vi "Test ACME SubTest.vi"(8 "error in (no error)":errorcluster, 11 "Label (VI Title)":string) -> (0 "error out":errorcluster)   [LabVIEW 2020]
uses:
  classes/Test/Test.lvclass
  Assert.ACME.lvclass
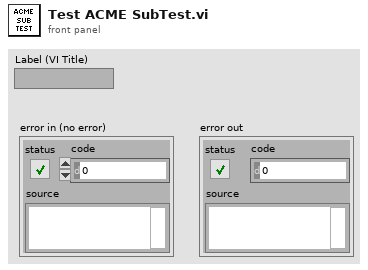
[diagram p1: front panel]
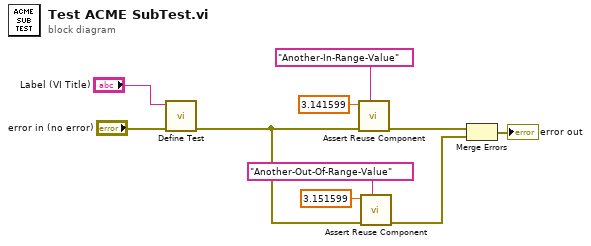
[diagram p0: block diagram]
diagram:
  n1 = call "Define Test.vi"("error in (no error)"="error in (no error)", "Label (VI Title)"="Label (VI Title)") -> ("error out"=w5:errorcluster)  [unwired: 8 in, 1 out]
  n2 = call "Assert Reuse Component.vi"("Label"="Another-In-Range-Value" ("Label (VI Title)"), "error in (no error)"=w5, "ACME Value"=3.141599) -> ("error out"=w9:errorcluster)  [unwired: 8 in]
  n3 = call "Assert Reuse Component.vi"("Label"="Another-Out-Of-Range-Value" ("Label (VI Title)"), "error in (no error)"=w5, "ACME Value"=3.151599) -> ("error out"=w3:errorcluster)  [unwired: 8 in]
  n4 = Merge Errors(w9, w3) -> (→"error out":errorcluster)
